vi "Drive Motor Set Speed.vi"(6 "Configuration":T2={"Accelerometer Bias"={"X (m/s)"=0.0, "Y (m/s)"=0.0, "Z (m/s)"=0.0}, "Gyroscope Bias"={"X (m/s)"=0.0, "Y (m/s)"=0.0, "Z (m/s)"=0.0}, "Steering Motor Gear Ratio"=611.0, "Steering Pully Gear Ratio"=1.0, "Steering Encoder CPR"=500.0, "Steering Motor Max RPM"=4000.0, "Wheelbase (m)"=1.12, "Fork Angle (rad)"=1.3, "Balancing Controller"={"Kp (/s)"=0.0, "Kd (1)"=0.0}, "Max Allowed Steering Angle (rad)"=0.7, "Task Periods"={"Emergency Stop (us)"=0, "IMU (us)"=0, "Steering Motor Encoder (us)"=0, "State Estimator (us)"=0, "Balancing Controller (us)"=0, "GNSS (us)"=0, "Logging (us)"=0, "Drive Motor (us)"=0, "Visualization (us)"=100000}, "Drive Motor Gear Ratio"=0.7, "lr"=10.0, "lf"=0.5986, "lambda"=1.2217, "k1"=0.004472, "k2"=0.09678, "e1_max"=11.331, "Ad_t"=0.95971, "Bd_t"=0.01, "C_t"=2.20588, "D_t"=0.0, "Wheel radius"=0.311}, 9 "Angular Speed (rad/s)":dbl, 10 "Drive Motor Handle In":T1, 11 "Error In":errorcluster) -> (2 "Drive Motor Handle Out":T1, 3 "Error Out":errorcluster)   [LabVIEW 2021]
uses:
  Drive Motor Handle.ctl
  Configuration/Configuration.ctl
panel:
  out "String":string
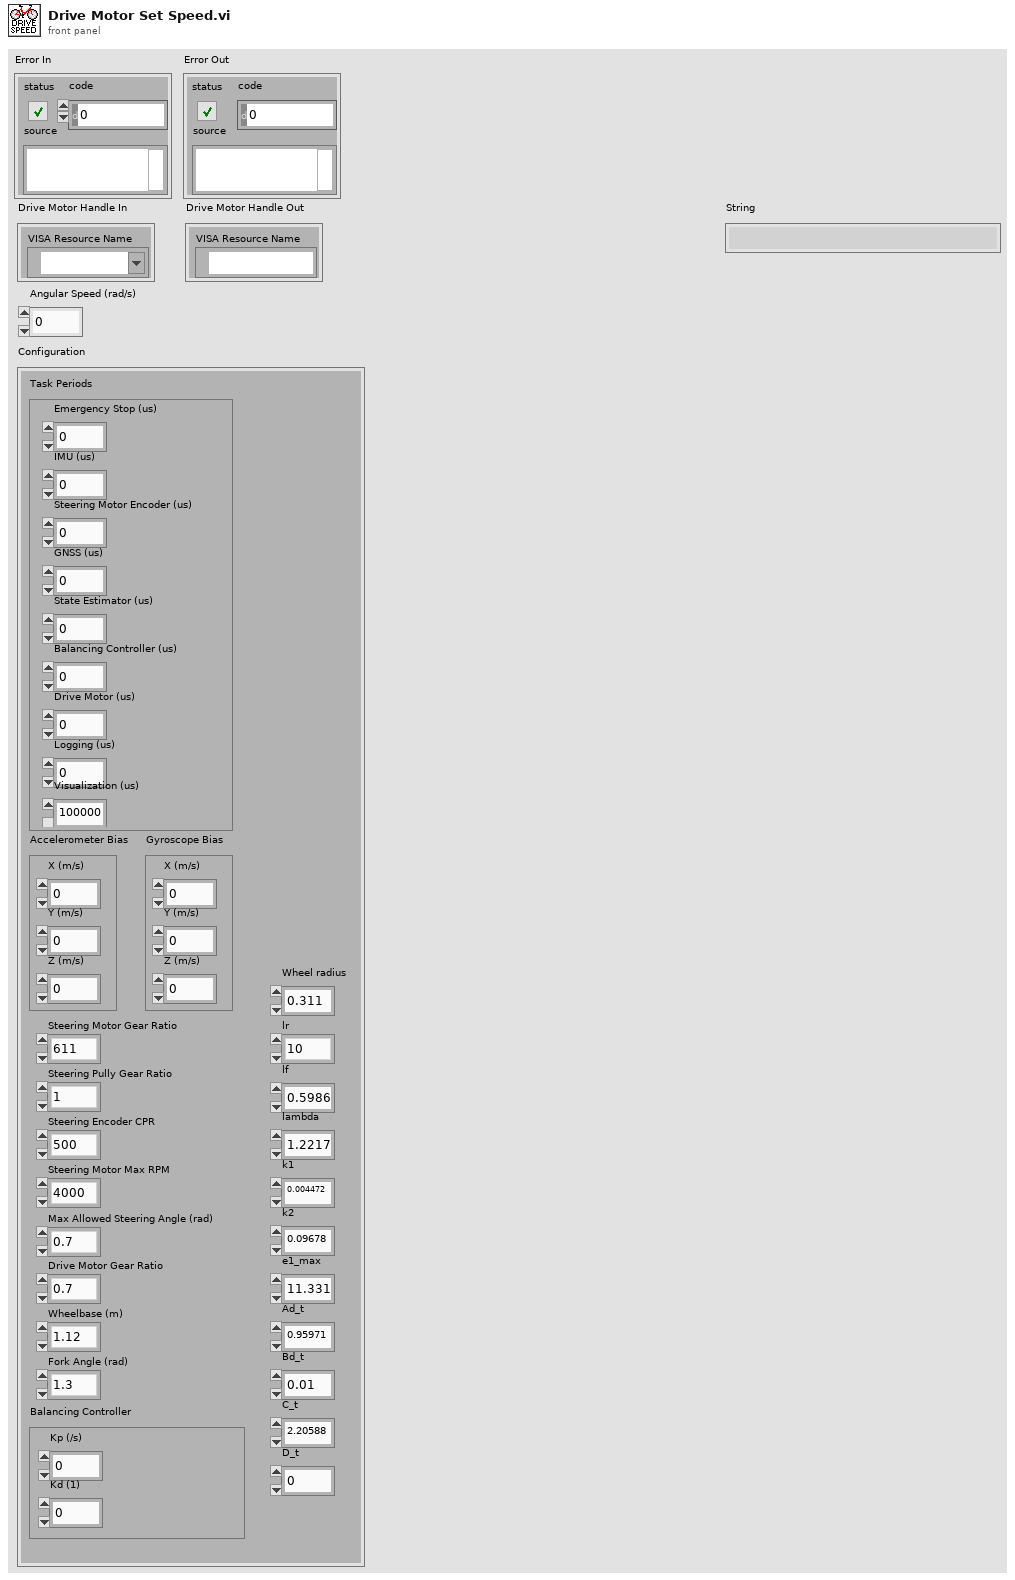
[diagram p1: front panel]
types:
  T1 = typedef "Drive Motor Handle.ctl" = cluster{"VISA Resource Name":refnum<visa-resource-name>}
  T2 = typedef "Configuration.ctl" = cluster{"Accelerometer Bias":cluster{"X (m/s)":dbl, "Y (m/s)":dbl, "Z (m/s)":dbl}, "Gyroscope Bias":cluster{"X (m/s)":dbl, "Y (m/s)":dbl, "Z (m/s)":dbl}, "Steering Motor Gear Ratio":dbl, "Steering Pully Gear Ratio":dbl, "Steering Encoder CPR":dbl, "Steering Motor Max RPM":dbl, "Wheelbase (m)":dbl, "Fork Angle (rad)":dbl, "Balancing Controller":cluster{"Kp (/s)":dbl, "Kd (1)":dbl}, "Max Allowed Steering Angle (rad)":dbl, "Task Periods":cluster{"Emergency Stop (us)":i64, "IMU (us)":i64, "Steering Motor Encoder (us)":i64, "State Estimator (us)":i64, "Balancing Controller (us)":i64, "GNSS (us)":i64, "Logging (us)":i64, "Drive Motor (us)":i64, "Visualization (us)":i64}, "Drive Motor Gear Ratio":dbl, "lr":dbl, "lf":dbl, "lambda":dbl, "k1":dbl, "k2":dbl, "e1_max":dbl, "Ad_t":dbl, "Bd_t":dbl, "C_t":dbl, "D_t":dbl, "Wheel radius":dbl}
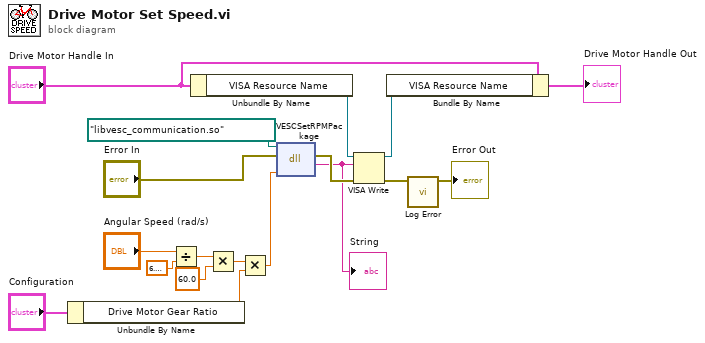
[diagram p0: block diagram]
diagram:
  n1 = Unbundle By Name("Configuration") -> ("Drive Motor Gear Ratio"=w9:dbl)
  n2 = Divide(x="Angular Speed (rad/s)", y=6.283185307179586) -> (x/y=w14:dbl)
  n3 = Unbundle By Name("Drive Motor Handle In") -> ("VISA Resource Name"=w5:refnum<visa-resource-name>)
  n4 = Multiply(x=w14, y=60.0) -> (x*y=w12:dbl)
  n5 = Multiply(x=w12, y=w9) -> (x*y=w11:dbl)
  n6 = dll-call lib="?" fn="VESCSetRPMPackage"(path in=path "libvesc_communication.so", error in="Error In", "RPM"=w11) -> (error out=w7:errorcluster, "Package"=w1:string)  [unwired: 2 in, 1 out]
  "String" <- w1
  n7 = VISA Write(VISA resource name=w5, write buffer=w1, error in (no error)=w7) -> (VISA resource name out=w4:refnum<visa-resource-name>, error out=w6:errorcluster)  [unwired: 1 out]
  n8 = Bundle By Name(cluster="Drive Motor Handle In", "VISA Resource Name"=w4) -> (→"Drive Motor Handle Out":T1)
  n9 = call "Log Error.vi"("Error In"=w6) -> ("Error Out"=→"Error Out":errorcluster)  [unwired: 10 in]
